vi "Get Sheets.vi"(8 "error in (no error)":errorcluster, 11 "Workbook Reference":refnum<k24>) -> (0 "error out":errorcluster, 3 "Workbook Reference":refnum<k24>, 4 "Sheets":string[](array[string]), 5 "NumberOfSheets":i32)   [LabVIEW 2013]
uses:
  C:/PhaeronGit/LVNPOI/Resources/NPOI 2.1.1 dotnet2/NPOI.dll
  Resources/NPOI 2.1.1 dotnet2/NPOI.dll
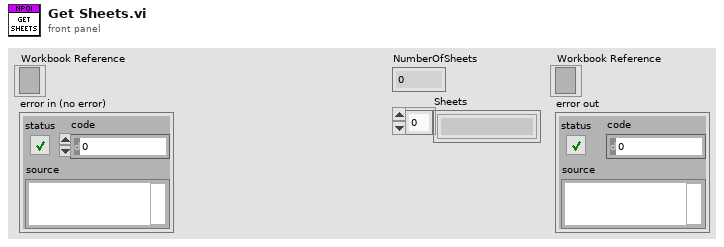
[diagram p1: front panel]
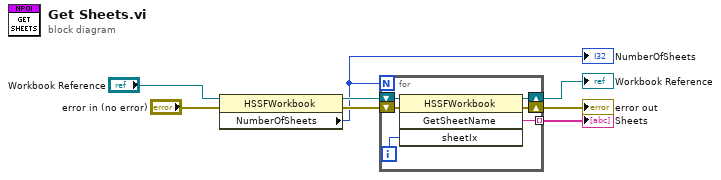
[diagram p0: block diagram]
diagram:
  n1 = property class="HSSFWorkbook"(reference="Workbook Reference", error in="error in (no error)") -> (reference out=w3:refnum<k24>, error out=w4:errorcluster, "NumberOfSheets"=w1:i32)
  "NumberOfSheets" <- w1
  n2 = for {
    N: w1 -> [_]
    shift-right: [w14] -> w8
    shift-left: w3 -> [w11]
    shift-right: [w13] -> w7
    shift-left: w4 -> [w12]
    tunnel: [w9] -> w2 mode=indexing
    i -> [w10]
    n3 = invoke class="HSSFWorkbook" method="GetSheetName"(reference=w11, error in=w12, "sheetIx"=w10) -> (reference out=w14:refnum<k24>, error out=w13:errorcluster, "GetSheetName"=w9:string)  [unwired: 1 in, 1 out]
  }
  "Workbook Reference" <- w8
  "error out" <- w7
  "Sheets" <- w2
